vi "selectScanTrigger.vi"(3 "scanTriggerEdge":T1=enum."true-false", 4 "MCSSelectScanTrigger":T2, 5 "triggerReadout":u16) -> (1 "fired":bool)   [LabVIEW 2014]
uses:
  Controls/selectTrigger.ctl
  Controls/triggerEdge.ctl
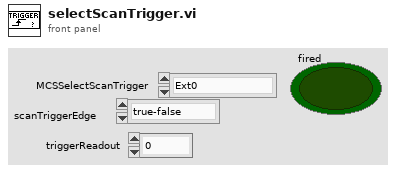
[diagram p1: front panel]
types:
  T1 = typedef "triggerEdge.ctl" = enum8{"either", "false-true", "true-false"}
  T2 = typedef "selectTrigger.ctl" = enum8{"Ext0", "Ext1", "Ext2", "Ext3", "Ext4", "Ext5", "Ext6", "Ext7", "Int0", "Int1", "Int2", "Int3", "Int4", "Int5", "Int6", "Int7"}
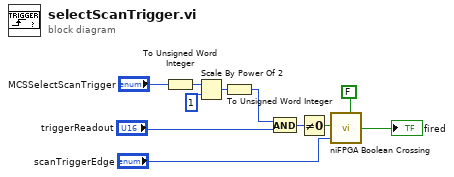
[diagram p0: block diagram]
diagram:
  n1 = To Unsigned Word Integer(number="MCSSelectScanTrigger") -> (unsigned 16bit integer=w7:u16)
  n2 = Scale By Power Of 2(n=w7, x=i16 1) -> (x*2^n=w5:i16)
  n3 = To Unsigned Word Integer(number=w5) -> (unsigned 16bit integer=w4:u16)
  n4 = And(x=w4, y="triggerReadout") -> (x .and. y?=w8:u16)
  n5 = Not Equal To 0?(x=w8) -> (x != 0?=w3:bool)
  n6 = call <vilib>:"niFPGA Boolean Crossing.vi"("input"=w3, "direction"="scanTriggerEdge", "initialize"=FALSE) -> ("crossing"=→"fired":bool)  [unwired: 6 in]
